vi "callback_userauth_publickey_sign_function.vi"(8 "error in (no error)":errorcluster, 10 "data":u8[](array[numeric])) -> (0 "error out":errorcluster, 2 "signature":u8[](array[numeric]))   [LabVIEW 2013, in "support.lvlib"]
doc: "Called when authenticating with libssh2 using <B>libssh2_userauth_publickey</B>.\n\n<B>data</B> data received from the remote server.\n<B>signature</B> signature for the data to authenticated on the server."
uses:
  support.lvlib
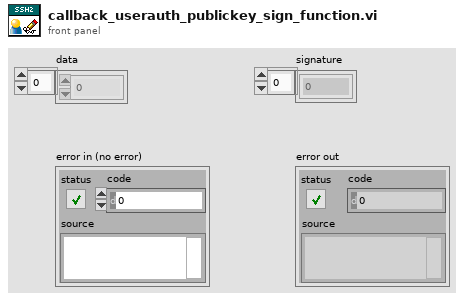
[diagram p1: front panel]
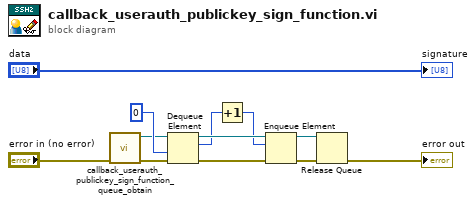
[diagram p0: block diagram]
diagram:
  n1 = call "callback_userauth_publickey_sign_function_queue_obtain.vi"("error in (no error)"="error in (no error)") -> ("error out"=w3:errorcluster, "queue out"=w4:refnum<queue>)  [unwired: 9 in]
  n2 = Dequeue Element(queue=w4, timeout in ms (-1)=0, error in (no error)=w3) -> (queue out=w7:refnum<queue>, element=w6:i64, error out=w11:errorcluster)  [unwired: 1 out]
  n3 = Increment(x=w6) -> (x+1=w5:i64)
  n4 = Enqueue Element(queue=w7, element=w5, error in (no error)=w11) -> (queue out=w8:refnum<queue>, error out=w9:errorcluster)  [unwired: 1 in, 1 out]
  n5 = Release Queue(queue=w8, error in (no error)=w9) -> (error out=→"error out":errorcluster)  [unwired: 1 in, 2 out]
  "signature" <- "data"
